vi "TCP-Parse Address and Port.vi"(7 "Address in":string) -> (6 "Address":string, 8 "success":bool, 10 "Port":i32)   [LabVIEW 2020]
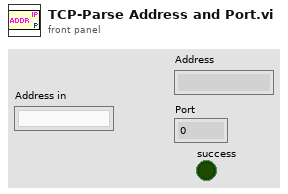
[diagram p1: front panel]
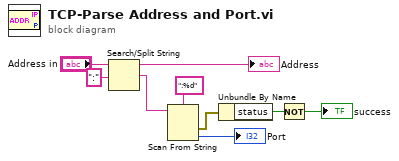
[diagram p0: block diagram]
diagram:
  n1 = Search/Split String(string="Address in", search string/char (-)=":") -> (substring before match=→"Address":string, match + rest of string=w3:string)  [unwired: 1 in, 1 out]
  n2 = Scan From String(format string=":%d", input string=w3) -> (error out=w8:errorcluster, output 1=→"Port":i32)  [unwired: 3 in, 2 out]
  n3 = Unbundle By Name(w8) -> ("status"=w7:bool)
  n4 = Not(x=w7) -> (.not. x?=→"success":bool)
